vi "Read Map - Center of Mass.vi"(11 "map":refnum<data-value>) -> (1 "Col":i32, 2 "Row":i32, 3 "map":refnum<data-value>)   [LabVIEW 2015, in "DS Square.lvlib"]
uses:
  DS Square.lvlib
  Square State.ctl
  Square Status.ctl
  Map.ctl
  Center of Mass.ctl
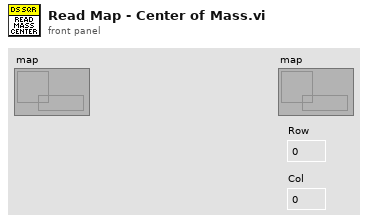
[diagram p1: front panel]
types:
  T1 = typedef "DS Square.lvlib/Map.ctl" = cluster{"squares":T2[][], "center of mass":T4}
  T2 = typedef "DS Square.lvlib/Square Status.ctl" = cluster{"square state":T3, "probability":dbl, "last update":i32}
  T3 = typedef "DS Square.lvlib/Square State.ctl" = enum16{"Unknown", "Empty", "Occupied - Active", "Occupied - Cool Down", "Attacked", "Enemy", "Enemy Wall"}
  T4 = typedef "DS Square.lvlib/Center of Mass.ctl" = cluster{"row":dbl, "col":dbl, "mass":dbl}
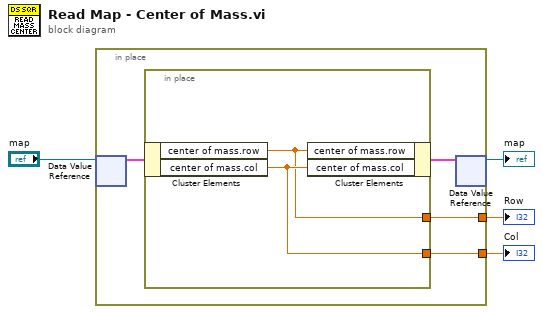
[diagram p0: block diagram]
diagram:
  n1 = in-place {
    in-place-border: [w6] -> w2
    in-place-border: [w5] -> w1
    n2 = in-place-dvr #1("map") -> (w8:T1)  [unwired: 1 out]
    n3 = in-place {
      in-place-border: [w10] -> w6
      in-place-border: [w9] -> w5
      n4 = in-place-cluster #2(w8) -> ("center of mass.row"=w9:dbl, "center of mass.col"=w10:dbl)
      n5 = in-place-cluster #2("center of mass.row"=w9, "center of mass.col"=w10) -> (w7:T1)
    }
    n6 = in-place-dvr #1(w7) -> (→"map":refnum<data-value>)  [unwired: 1 out]
  }
  "Row" <- w1
  "Col" <- w2
